vi "Write Product Name.vi"(8 "error in (no error)":errorcluster, 10 "Product Name":string, 11 "Component in":refnum<class "Component.lvclass">) -> (0 "error out":errorcluster, 3 "Component out":refnum<class "Component.lvclass">)   [LabVIEW 2017, in "CL_G3_VIComponentBuilder.lvlib" / "Component.lvclass"]
uses:
  Component.lvclass
  Component.lvclass/Component.ctl
  Read Component Config File.vi
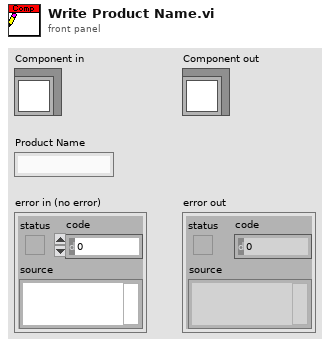
[diagram p1: front panel]
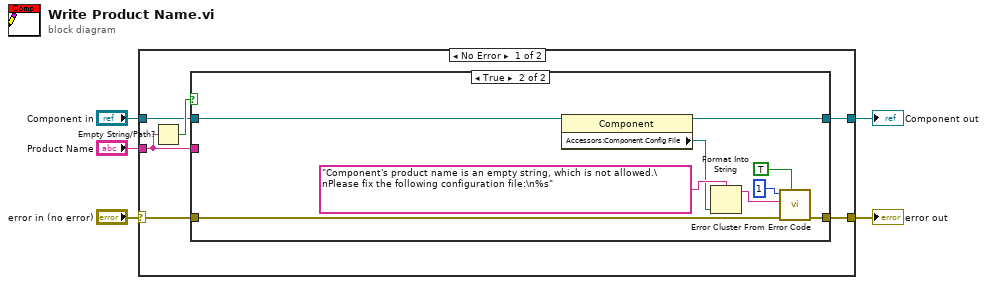
[diagram p0: block diagram]
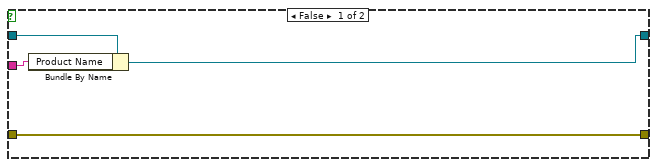
[diagram p2: hidden frame]
diagram:
  n1 = case shown="No Error" "error in (no error)" {
    selector: "error in (no error)" -> [w8 w25]
    tunnel: [w9 w25] -> w4
    tunnel: [w6 w26] -> w2
    tunnel: "Component in" -> [w10 w26]
    tunnel: "Product Name" -> [w7 _]
    frame No Error {
      n2 = Empty String/Path?(string/path=w7) -> (empty?=w11:bool)
      n3 = case shown="True" w11 {
        tunnel: w8 -> [w15 w23]
        tunnel: [w15 w16] -> w9
        tunnel: w10 -> [w14 w24]
        tunnel: [w13 w17] -> w6
        tunnel: w7 -> [w12 _]
        frame False {
          n4 = Bundle By Name(cluster=w14, "Product Name"=w12) -> (w13:refnum<class "Component.lvclass">)
        }
        frame True {
          n5 = property class="Component"(reference=w24) -> (reference out=w17:refnum<class "Component.lvclass">, "Accessors:Component Config File"=w19:path)  [unwired: 1 in, 1 out]
          n6 = Format Into String(format string="Component's product name is an empty string, which is not allowed.\nPlease fix the following configuration file:\n%s" ("error message (\"\")"), w19) -> (resulting string=w18:string)  [unwired: 2 in, 1 out]
          n7 = call <vilib>:"Error Cluster From Error Code.vi"("show call chain? (False)"=TRUE, "error in (no error)"=w23, "error message (\"\")"=w18, "error code (0)"=1) -> ("error out"=w16:errorcluster)  [unwired: 5 in]
        }
      }
    }
    frame Error {
    }
  }
  "error out" <- w4
  "Component out" <- w2
